vi "HEIGHT.vi"() -> (0 "HEIGHT":i16=300)   [LabVIEW 2020]
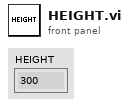
[diagram p1: front panel]
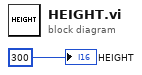
[diagram p0: block diagram]
diagram:
  "HEIGHT" <- i16 300
